vi "Cryo-Con -- Get T.vi"(8 "error in (no error)":errorcluster, 10 "Channel":string="A", 11 "VISA Resource Name":refnum<visa-resource-name>) -> (0 "error out":errorcluster, 1 "data string":string, 2 "Temperature":dbl format="%.5f", 3 "VISA Resource Name Out":refnum<visa-resource-name>)   [LabVIEW 2017]
uses:
  NHMFL_Core/Libraries/Instruments/GPIB/VISA  Send Receive.vi
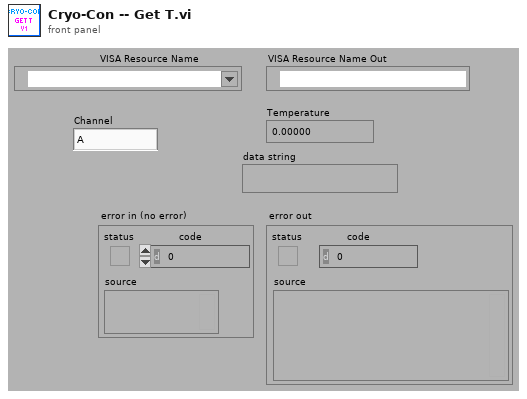
[diagram p1: front panel]
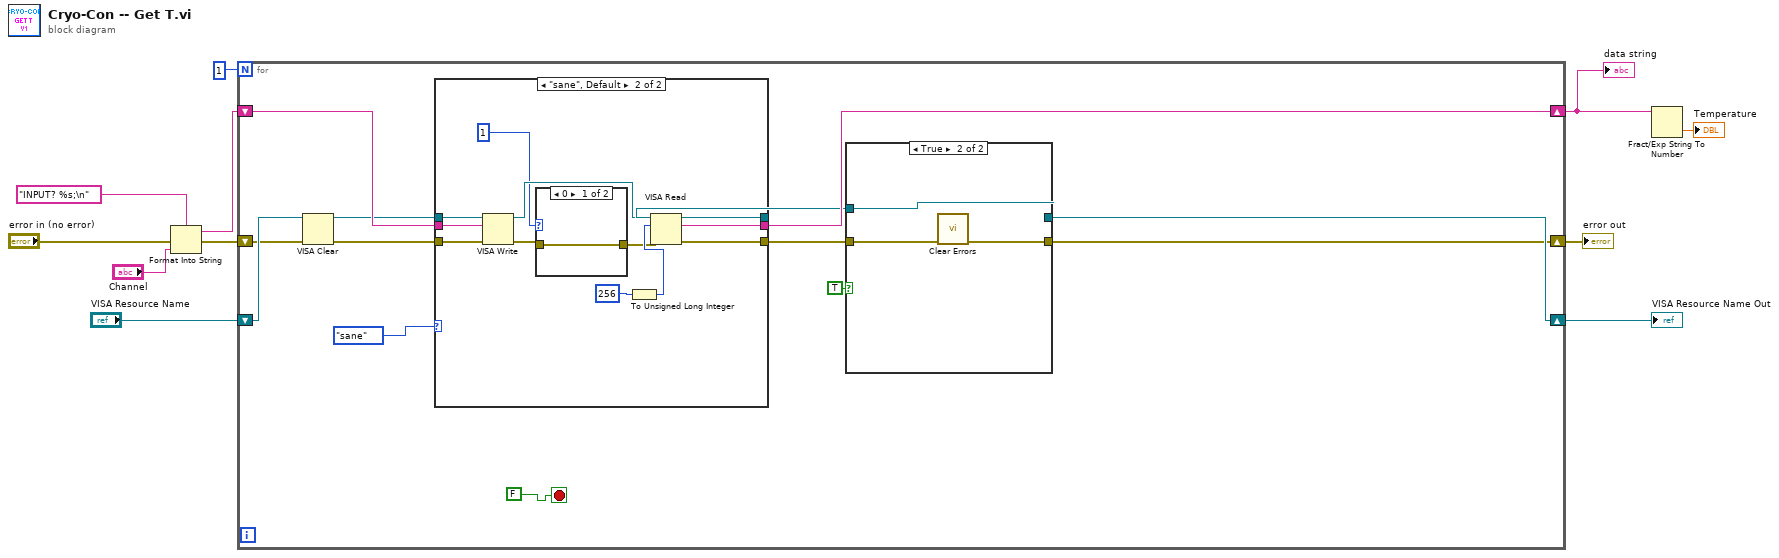
[diagram p0: block diagram]
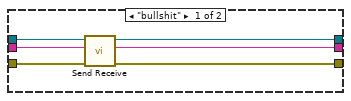
[diagram p2: hidden frame]
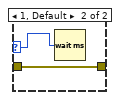
[diagram p3: hidden frame]
diagram:
  n1 = Format Into String(format string="INPUT? %s;\n" ("data string"), error in="error in (no error)", "Channel") -> (resulting string=w5:string, error out=w6:errorcluster)  [unwired: 1 in]
  n2 = for {
    N: 1 -> [_]
    shift-right: [w21] -> w9
    shift-left: "VISA Resource Name" -> [w18]
    shift-right: [w19] -> w11
    shift-left: w6 -> [w16]
    shift-right: [w23] -> w4
    shift-left: w5 -> [w24]
    stop <- FALSE stop-if-true
    n3 = VISA Clear(VISA resource name=w18, error in (no error)=w16) -> (VISA resource name out=w17:refnum<visa-resource-name>, error out=w15:errorcluster)
    n4 = case shown="\"sane\", Default" enum16{"sane", "bullshit"}."sane" {
      tunnel: w24 -> [w30 w38]
      tunnel: [w29 w37] -> w23
      tunnel: [w28 w41] -> w22
      tunnel: [w27 w39] -> w20
      tunnel: w17 -> [w26 w42]
      tunnel: w15 -> [w25 w40]
      frame "bullshit" {
        n5 = call-poly "Send Receive.vi"("error in (no error)"=w25, "data string in"=w30, "VISA Resource Name"=w26) -> ("error out"=w27:errorcluster, "data string out"=w29:string, "VISA Resource Name Out"=w28:refnum<visa-resource-name>)  [unwired: 6 in]
      }
      frame "sane", Default {
        n6 = VISA Write(VISA resource name=w42, write buffer=w38, error in (no error)=w40) -> (VISA resource name out=w32:refnum<visa-resource-name>, error out=w34:errorcluster)  [unwired: 1 out]
        n7 = case shown="0" u32 1 ("Read Delay, ms") {
          selector: u32 1 ("Read Delay, ms") -> [_ w44]
          tunnel: w34 -> [w43 w45]
          tunnel: [w43 w45] -> w33
          frame 0 {
          }
          frame 1, Default {
            n8 = Wait (ms)(milliseconds to wait=w44) -> ()  [unwired: 1 out]
          }
        }
        n9 = To Unsigned Long Integer(number=u32 256 ("byte count")) -> (unsigned 32bit integer=w35:u32)
        n10 = VISA Read(VISA resource name=w32, byte count=w35, error in (no error)=w33) -> (VISA resource name out=w41:refnum<visa-resource-name>, read buffer=w37:string, error out=w39:errorcluster)  [unwired: 1 out]
      }
    }
    n11 = case shown="True" TRUE {
      tunnel: w20 -> [w47 w50]
      tunnel: w22 -> [w46 w48]
      tunnel: [w47 w49] -> w19
      tunnel: [w46 w48] -> w21
      frame False {
      }
      frame True {
        n12 = call <vilib>:"Clear Errors.vi"("error in (no error)"=w50) -> ("error out"=w49:errorcluster)  [unwired: 5 in, 1 out]
      }
    }
  }
  "error out" <- w11
  "data string" <- w4
  "VISA Resource Name Out" <- w9
  n13 = Fract/Exp String To Number(string=w4) -> (number=→"Temperature":dbl)  [unwired: 4 out]
